vi "test_No Instrument Addon Found.vi"(8 "error in (no error)":errorcluster, 11 "TestCase in":refnum<class "Instrument Addon Scripting API Custom Device Unit Tests.lvclass">) -> (0 "error out":errorcluster, 3 "TestCase out":refnum<class "Instrument Addon Scripting API Custom Device Unit Tests.lvclass">)   [LabVIEW 2018, in "Instrument Addon Scripting API Custom Device Unit Tests.lvclass"]
uses:
  Instrument Addon Scripting API Custom Device Unit Tests.lvclass
  <vilib>/addons/_JKI Toolkits/VI Tester/TestCase.llb/TestCase.lvclass
  Instrument Addon Scripting API Test Assets/Instrument Addon Scripting API Test Assets.lvclass
  APIs/Scripting API/Instrument Addon Scripting API.lvlib
  C:/Program Files (x86)/National Instruments/LabVIEW 2018/vi.lib/addons/_JKI Toolkits/VI Tester/TestCase.llb/TestCase.lvclass
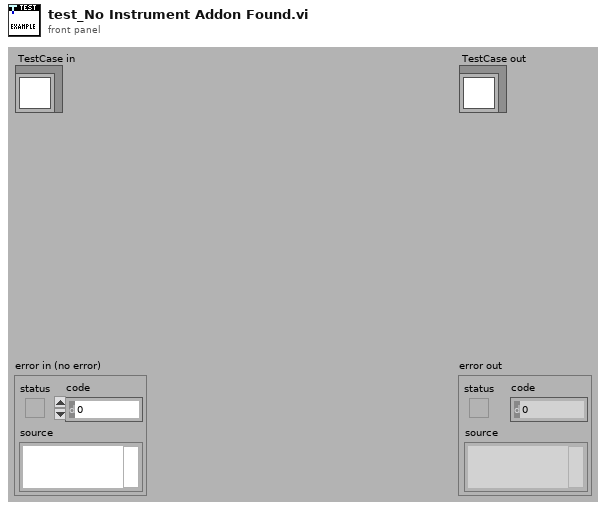
[diagram p1: front panel]
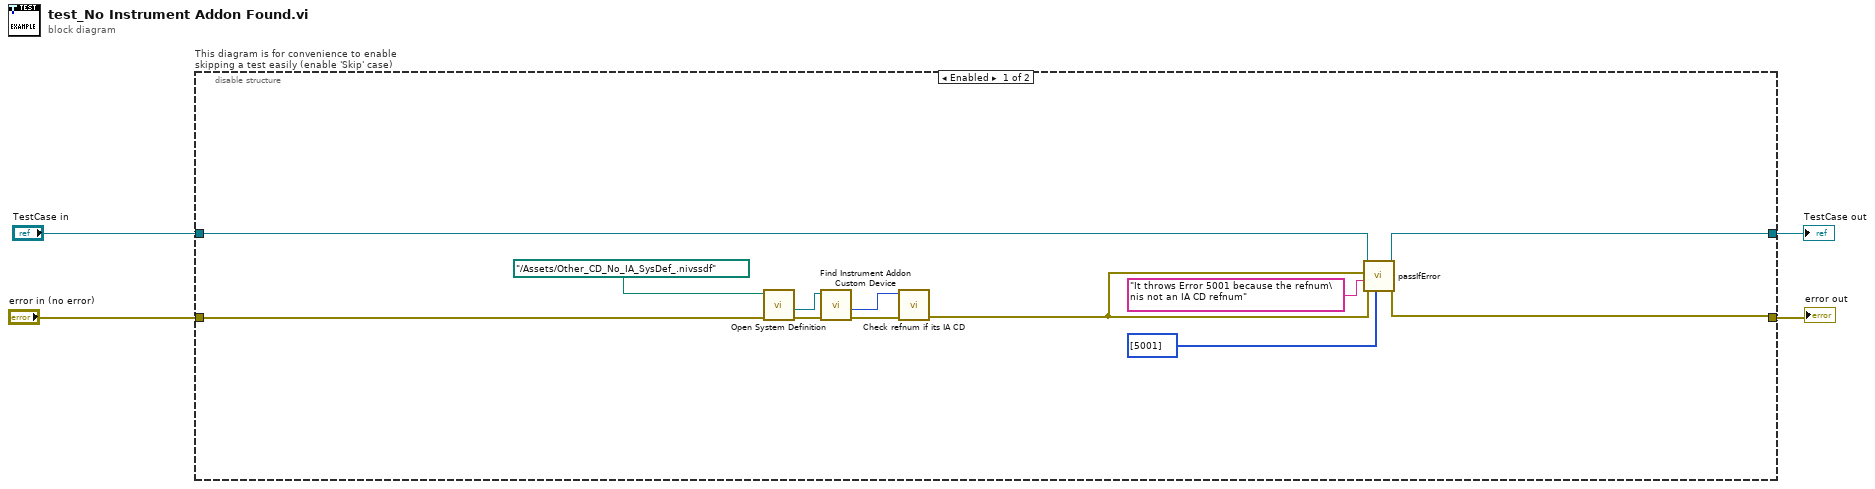
[diagram p0: block diagram]
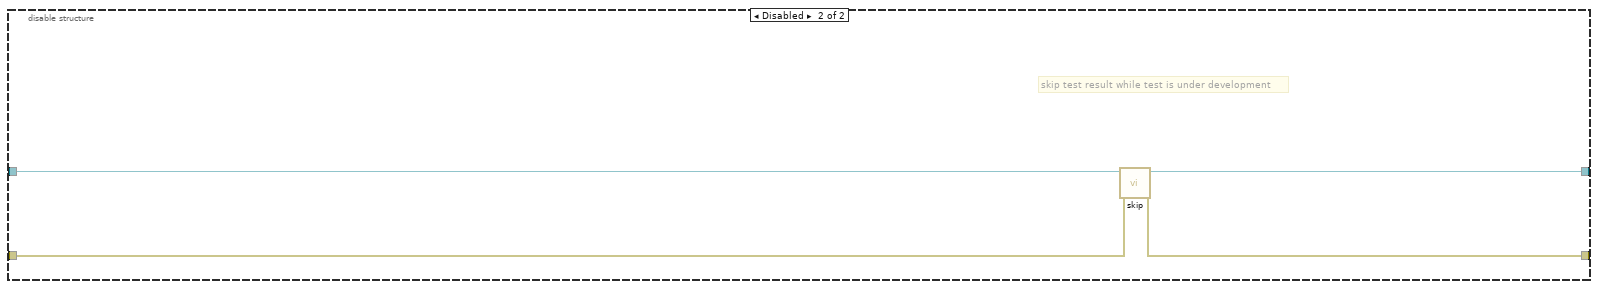
[diagram p2: hidden frame]
diagram:
  n1 = disable-structure "This diagram is for convenience to enable skipping a test easily (enable 'Skip' case)" shown="Enabled" {
    disable-tunnel: "TestCase in" -> [w16 w20]
    disable-tunnel: [w15 w18] -> w1
    disable-tunnel: [w14 w19] -> w3
    disable-tunnel: "error in (no error)" -> [w13 w17]
    frame Enabled {
      n2 = call "Open System Definition.vi"("error in (no error)"=w13, "System Definition File"=path "../Assets/Other_CD_No_IA_SysDef_.nivssdf") -> ("error out"=w12:errorcluster, "Target Refnum"=w11:refnum<k24>)  [unwired: 6 in, 2 out]
      n3 = call "Find Instrument Addon Custom Device.vi"("error in"=w12, "target in"=w11) -> ("error out"=w8:errorcluster, "NodeID"=w5:u64)  [unwired: 7 in, 1 out]
      n4 = call "Check refnum if its IA CD.vi"("Error In"=w8, "Refnum In"=w5) -> ("Error Out"=w7:errorcluster)  [unwired: 7 in, 2 out]
      n5 = call-dynamic "passIfError.vi"("passing error codes (default = any error code)"=i32[] [5001], "error in (no error)"=w7, "task (\"\")"="It throws Error 5001 because the refnum\nis not an IA CD refnum" ("task (\"\")"), "error"=w7, "TestCase in"=w16) -> ("error out"=w14:errorcluster, "TestCase out"=w15:refnum<class "Instrument Addon Scripting API Custom Device Unit Tests.lvclass">)  [unwired: 5 in]
    }
    frame Disabled {
      # "skip test result while test is under development"
      n6 = call <vilib>:"skip.vi"("error in (no error)"=w17, "TestCase in"=w20) -> ("error out"=w19:errorcluster, "TestCase out"=w18:refnum<class "Instrument Addon Scripting API Custom Device Unit Tests.lvclass">)  [unwired: 8 in]
    }
  }
  "error out" <- w3
  "TestCase out" <- w1
